vi "Configure Controls.vi"(8 "error in":errorcluster, 11 "TEC Controller in":refnum<class "TEC Controller.lvclass">) -> (0 "error out":errorcluster, 3 "TEC Controller out":refnum<class "TEC Controller.lvclass">)   [LabVIEW 2014, in "Humidifier Test Lib.lvlib" / "TEC Controller.lvclass"]
uses:
  TEC Controller.lvclass
  reusable/Session APIs/File Access/Config Data/Config Data.lvclass
  TEC Controller.lvclass/TEC Controller.ctl
  reusable/Session APIs/File Access/Config Data/Config Data.lvclass/Config Data.ctl
  reusable/Session APIs/File Access/Config Data/Accessors/Read Ref.vi
  <vilib>/Utility/config.llb/Read Key (Double).vi
  <vilib>/Utility/config.llb/Read Key (Boolean).vi
  <vilib>/Utility/config.llb/NI_LVConfig.lvlib
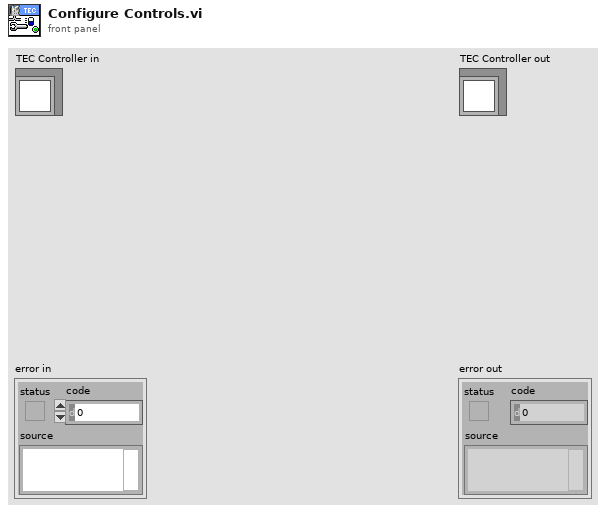
[diagram p1: front panel]
types:
  T1 = typedef "Session - Root.lvclass/Session Handle.ctl" = refnum<data-value>
  T2 = typedef "NI_LVConfig.lvlib/Config Data RefNum.ctl" = refnum<k1>
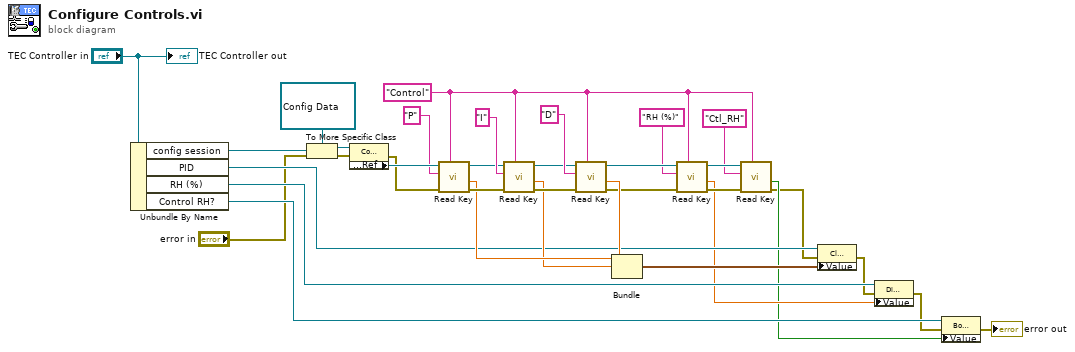
[diagram p0: block diagram]
diagram:
  w17 = "Control" ("section")
  n1 = Unbundle By Name("TEC Controller in") -> ("config session"=w35:T1, "PID"=w13:refnum<vi>, "RH (%)"=w11:refnum<vi>, "Control RH?"=w9:refnum<vi>)
  n2 = To More Specific Class(target class=refnum<data-value> refnum, reference=w35, error in="error in") -> (specific class reference=w33:refnum<data-value>, error out=w14:errorcluster)
  n3 = property class="Config Data"(reference=w33, error in=w14) -> (error out=w6:errorcluster, "Accessors:Ref"=w32:T2)  [unwired: 1 out]
  n4 = call-poly <vilib>:"Read Key.vi"("section"=w17, "error in (no error)"=w6, "key"="P", "refnum"=w32) -> ("error out"=w28:errorcluster, "value"=w24:dbl, "refnum out"=w29:T2)  [unwired: 4 in, 1 out]
  n5 = call-poly <vilib>:"Read Key.vi"("section"=w17, "error in (no error)"=w28, "key"="I", "refnum"=w29) -> ("error out"=w25:errorcluster, "value"=w23:dbl, "refnum out"=w26:T2)  [unwired: 4 in, 1 out]
  n6 = call-poly <vilib>:"Read Key.vi"("section"=w17, "error in (no error)"=w25, "key"="D", "refnum"=w26) -> ("error out"=w20:errorcluster, "value"=w22:dbl, "refnum out"=w21:T2)  [unwired: 4 in, 1 out]
  n7 = Bundle("value"=w24, "value"=w23, "value"=w22) -> (w12:cluster{"value":dbl, "value":dbl, "value":dbl})  [unwired: 1 in]
  n8 = call-poly <vilib>:"Read Key.vi"("section"=w17, "error in (no error)"=w20, "key"="RH (%)", "refnum"=w21) -> ("error out"=w16:errorcluster, "value"=w10:dbl, "refnum out"=w18:T2)  [unwired: 4 in, 1 out]
  n9 = call-poly <vilib>:"Read Key.vi"("section"=w17, "error in (no error)"=w16, "key"="Ctl_RH", "refnum"=w18) -> ("error out"=w4:errorcluster, "value"=w8:bool)  [unwired: 4 in, 2 out]
  n10 = property class="Clust (strict)"(reference=w13, error in=w4, "Value"=w12) -> (error out=w3:errorcluster)  [unwired: 1 out]
  n11 = property class="DigNum (strict)"(reference=w11, error in=w3, "Value"=w10) -> (error out=w2:errorcluster)  [unwired: 1 out]
  n12 = property class="Bool (strict)"(reference=w9, error in=w2, "Value"=w8) -> (error out=→"error out":errorcluster)  [unwired: 1 out]
  "TEC Controller out" <- "TEC Controller in"
